vi "CLD 13 Flow Rate Calculations.vi"(8 "Error In":errorcluster, 11 "Cluster in":T1) -> (0 "Error Out":errorcluster, 3 "Cluster out":T1)   [LabVIEW 2018]
doc: "CLD 13 Logic for changing the flow rate. The algorithm takes single value steps when the rate is near zero. This simplifies the elapsed time function."
uses:
  CLD 13 Data Cluster.ctl
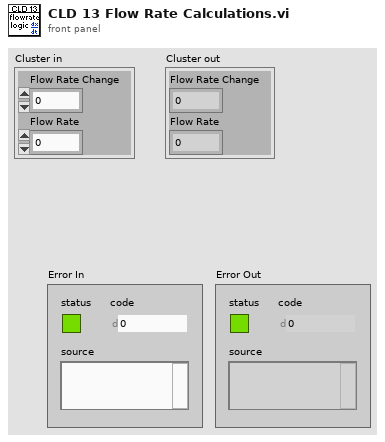
[diagram p1: front panel]
types:
  T1 = typedef "CLD 13 Data Cluster.ctl" = cluster{"Flow Rate Change":i8, "Flow Rate":i8}
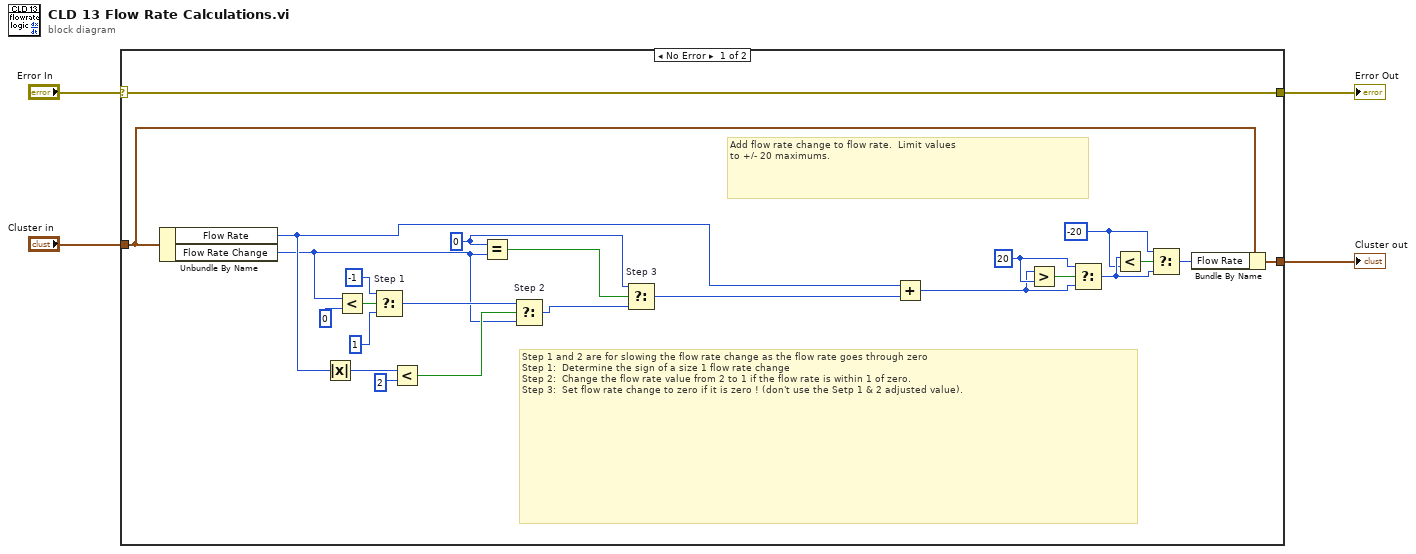
[diagram p0: block diagram]
diagram:
  n1 = case shown="No Error" "Error In" {
    selector: "Error In" -> [w5 w30]
    tunnel: [w20 w29] -> w4
    tunnel: "Cluster in" -> [w18 w29]
    tunnel: [w5 w30] -> w1
    frame No Error {
      w27 = i8 0 ("x")
      w16 = i8 -20 ("y")
      w14 = i8 20 ("y")
      # "Add flow rate change to flow rate.  Limit values \nto +/- 20 maximums."
      # "Step 1 and 2 are for slowing the flow rate change as the flow rate goes through zero \nStep 1:  Determine the sign of a size 1 flow rate change\nStep 2:  Change the flow rate value from 2 to 1 if the flow rate is within 1 of zero.\nStep 3:  Set flow rate change to zero if it is zero ! (don't use the Setp 1 & 2 adjusted value)."
      n2 = Unbundle By Name(w18) -> ("Flow Rate"=w8:i8, "Flow Rate Change"=w7:i8)
      n3 = Absolute Value(x=w8) -> (abs(x)=w10:i8)
      n4 = Less?(x=w7, y=i8 0 ("x")) -> (x < y?=w22:bool)
      n5 = Select "Step 1"(t=i8 -1, s=w22, f=i8 1 ("t")) -> (s? t:f=w25:i8)
      n6 = Less?(x=w10, y=i8 2) -> (x < y?=w11:bool)
      n7 = Equal?(x=w27, y=w7) -> (x = y?=w26:bool)
      n8 = Select "Step 2"(t=w25, s=w11, f=w7) -> (s? t:f=w28:i8)
      n9 = Select "Step 3"(t=w27, s=w26, f=w28) -> (s? t:f=w6:i8)
      n10 = Add(x=w8, y=w6) -> (x+y=w13:i8)
      n11 = Greater?(x=w13, y=w14) -> (0:w12:bool)
      n12 = Select(t=w14, s=w12, f=w13) -> (s? t:f=w17:i8)
      n13 = Less?(x=w17, y=w16) -> (x < y?=w15:bool)
      n14 = Select(t=w16, s=w15, f=w17) -> (s? t:f=w19:i8)
      n15 = Bundle By Name(cluster=w18, "Flow Rate"=w19) -> (w20:T1)
    }
    frame Error {
    }
  }
  "Cluster out" <- w4
  "Error Out" <- w1
